vi "Name.vi"(11 "No Popup Data Type in":refnum<class "No Popup Data Type.lvclass">) -> (2 "String":string="Generic", 3 "No Popup Data Type (dup)":refnum<class "No Popup Data Type.lvclass">)   [LabVIEW 2018, in "No Popup Data Type.lvclass"]
uses:
  No Popup Data Type.lvclass
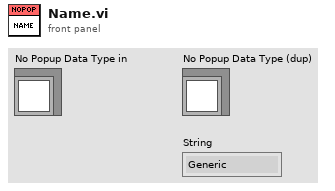
[diagram p1: front panel]
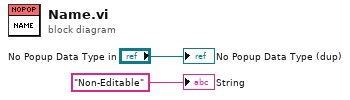
[diagram p0: block diagram]
diagram:
  "No Popup Data Type (dup)" <- "No Popup Data Type in"
  "String" <- "Non-Editable" ("String")
